vi "Frame Ready.vi"(8 "error in (no error)":errorcluster, 9 "Processed Frames per Second":dbl, 10 "Image In":T1, 11 "Camera_Controller in":refnum<class "Camera_Controller.lvclass">) -> (0 "error out":errorcluster, 3 "Camera_Controller out":refnum<class "Camera_Controller.lvclass">)   [LabVIEW 2023, in "Camera_Controller.lvlib" / "Camera_Controller.lvclass"]
uses:
  Camera_Controller.lvclass
  <vilib>/vision/Image Controls.llb/IMAQ Image.ctl
  Camera_Controller.lvclass/Camera_Controller.ctl
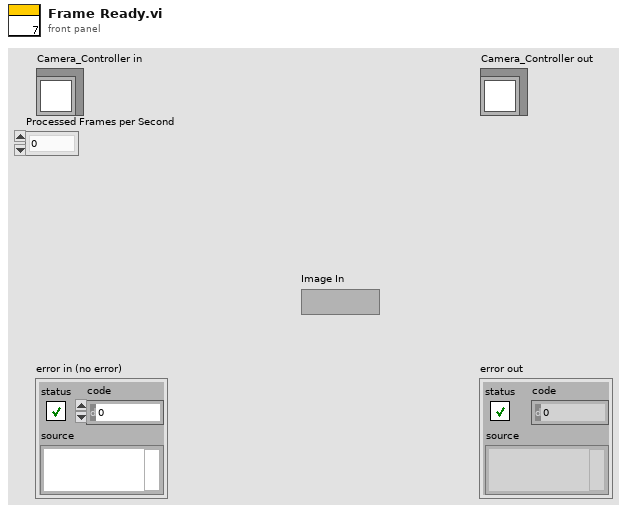
[diagram p1: front panel]
types:
  T1 = typedef "IMAQ Image.ctl" = refnum<image>
  T2 = cluster{"Image In":T1, "Processed Frames per Second":dbl}
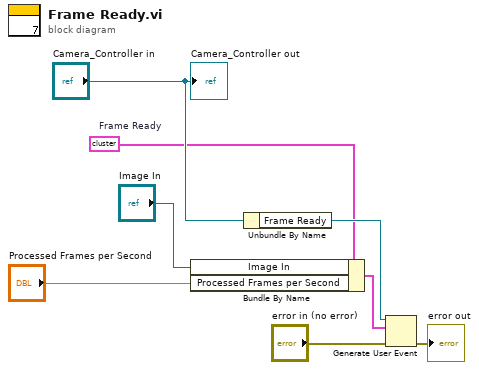
[diagram p0: block diagram]
diagram:
  w1 = T2 {"Image In"=refnum, "Processed Frames per Second"=0.0}  # Frame Ready
  n1 = Bundle By Name(cluster=w1, "Image In"="Image In", "Processed Frames per Second"="Processed Frames per Second") -> (w2:T2)
  n2 = Unbundle By Name("Camera_Controller in") -> ("Frame Ready"=w7:refnum<user-event>)
  n3 = Generate User Event(user event=w7, event data cluster=w2, error in="error in (no error)") -> (error out=→"error out":errorcluster)  [unwired: 1 in, 1 out]
  "Camera_Controller out" <- "Camera_Controller in"
